vi "RIOprime.vi"(8 "Error in":errorcluster, 10 "RIO Card/Channels":i32[](array[numeric]), 11 "Tree DVR in":refnum<data-value>) -> (0 "Error out":errorcluster)   [LabVIEW 2014]
uses:
  <vilib>/MDSplus/Classes/Tree_Class/Tree.lvclass
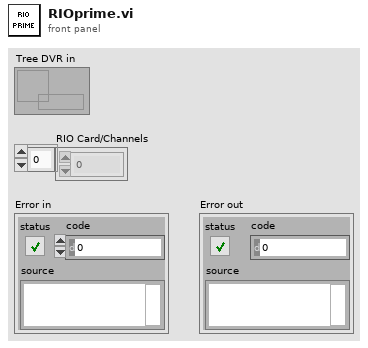
[diagram p1: front panel]
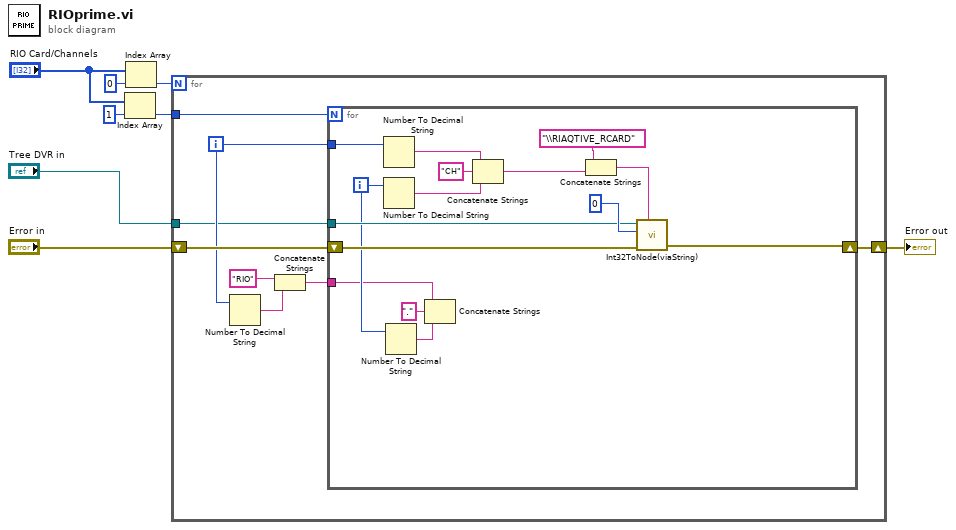
[diagram p0: block diagram]
diagram:
  n1 = Index Array(array="RIO Card/Channels", index=1) -> (element=w6:i32)
  n2 = Index Array(array="RIO Card/Channels", index=0) -> (element=w5:i32)
  n3 = for {
    N: w5 -> [_]
    shift-right: [w12] -> w4
    shift-left: "Error in" -> [w13]
    tunnel: w6 -> [w16]
    tunnel: "Tree DVR in" -> [w10]
    i -> [w11]
    n4 = Number To Decimal String(number=w11) -> (decimal integer string=w15:string)  [unwired: 1 in]
    n5 = Concatenate Strings("RIO", w15) -> (w9:string)
    n6 = for {
      N: w16 -> [_]
      shift-right: [w17] -> w12
      shift-left: w13 -> [w22]
      tunnel: w11 -> [w28]
      tunnel: w10 -> [w23]
      tunnel: w9 -> [w18]
      i -> [w19]
      n7 = Number To Decimal String(number=w28) -> (decimal integer string=w30:string)  [unwired: 1 in]
      n8 = Number To Decimal String(number=w19) -> (decimal integer string=w29:string)  [unwired: 1 in]
      n9 = Number To Decimal String(number=w19) -> (decimal integer string=w20:string)  [unwired: 1 in]
      n10 = Concatenate Strings(w18, "." ("string"), w20) -> ()  [unwired: 1 out]
      n11 = Concatenate Strings(w30, "CH" ("string"), w29) -> (w26:string)
      n12 = Concatenate Strings("\\RIAQTIVE_RCARD" ("string"), w26) -> (w24:string)
      n13 = call "Int32ToNode(viaString).vi"("Tree DVR in"=w23, "I32 in"=0, "error in (no error)"=w22, "NodePath"=w24) -> ("error out"=w17:errorcluster)  [unwired: 3 in]
    }
  }
  "Error out" <- w4
